vi "Configure DC Input Resistance.vi"(8 "error in (no error)":errorcluster, 10 "Auto Impedance (F: Disable)":bool, 11 "VISA resource name":refnum<visa-resource-name>) -> (0 "error out":errorcluster, 3 "VISA resource name out":refnum<visa-resource-name>)   [LabVIEW 2020, in "Agilent 34405.lvlib"]
doc: "Configures the automatic input impedance mode for dc voltage measurements.\n\n<B>Notes:</B>\n(1) This VI affects <B>DC Voltage</B> measurements only.\n(2) This VI only support <B>Agilent 34450A</B>."
uses:
  <instrlib>/Agilent 34405/Agilent 34405.lvlib
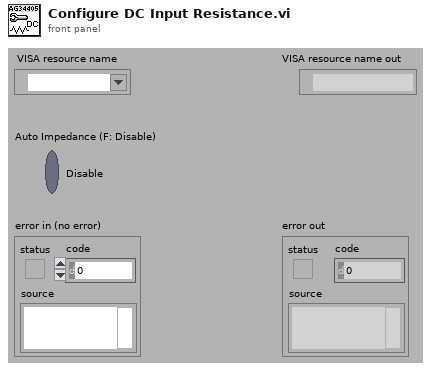
[diagram p1: front panel]
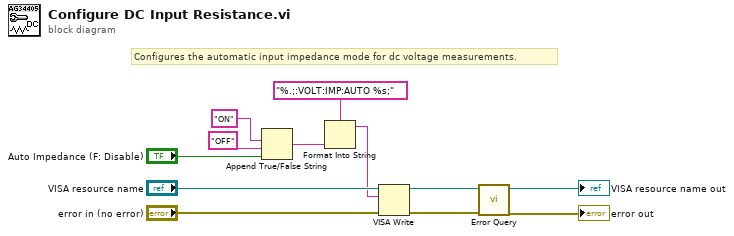
[diagram p0: block diagram]
diagram:
  # "Configures the automatic input impedance mode for dc voltage measurements."
  n1 = Append True/False String(1:"Auto Impedance (F: Disable)", 2:"OFF", 3:"ON") -> (0:w3:string)  [unwired: 1 out]
  n2 = Format Into String(format string="%.;:VOLT:IMP:AUTO %s;", w3) -> (resulting string=w2:string)  [unwired: 2 in, 1 out]
  n3 = VISA Write(VISA resource name="VISA resource name", write buffer=w2, error in (no error)="error in (no error)") -> (VISA resource name out=w10:refnum<visa-resource-name>, error out=w9:errorcluster)  [unwired: 1 out]
  n4 = call <instrlib>:"Error Query.vi"("error in (no error)"=w9, "VISA resource name"=w10) -> ("error out"=→"error out":errorcluster, "VISA resource name out"=→"VISA resource name out":refnum<visa-resource-name>)  [unwired: 8 out]
